vi "InitConnection.vi"(8 "ErrorIn":errorcluster) -> (0 "ErrorOut":errorcluster, 3 "Reference":T1)   [LabVIEW 2022 SP3]
uses:
  C:/Users/Robots/Documents/robocadSimLV/assemblies/LibraryForLabVIEW.dll
  assemblies/LibraryForLabVIEW.dll
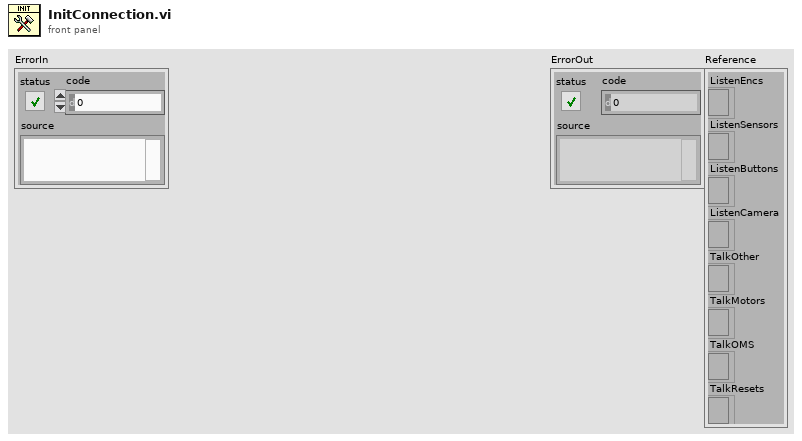
[diagram p1: front panel]
types:
  T1 = cluster{"ListenEncs":refnum<k24>, "ListenSensors":refnum<k24>, "ListenButtons":refnum<k24>, "ListenCamera":refnum<k24>, "TalkOther":refnum<k24>, "TalkMotors":refnum<k24>, "TalkOMS":refnum<k24>, "TalkResets":refnum<k24>}
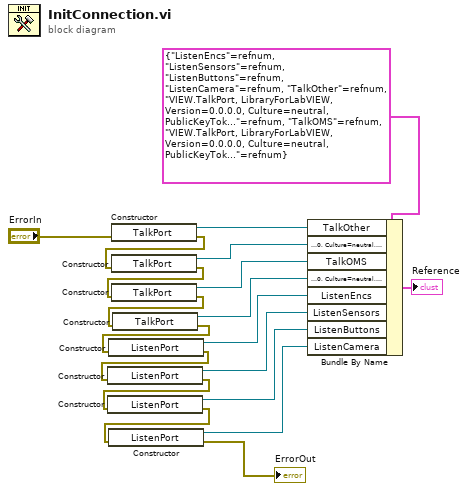
[diagram p0: block diagram]
diagram:
  n1 = constructor class="TalkPort"(error in="ErrorIn") -> (reference out=w17:refnum<k24>, error out=w15:errorcluster)  [unwired: 2 in, 1 out]
  n2 = constructor class="TalkPort"(error in=w15) -> (reference out=w16:refnum<k24>, error out=w13:errorcluster)  [unwired: 2 in, 1 out]
  n3 = constructor class="TalkPort"(error in=w13) -> (reference out=w14:refnum<k24>, error out=w11:errorcluster)  [unwired: 2 in, 1 out]
  n4 = constructor class="TalkPort"(error in=w11) -> (reference out=w12:refnum<k24>, error out=w9:errorcluster)  [unwired: 2 in, 1 out]
  n5 = constructor class="ListenPort"(error in=w9) -> (reference out=w10:refnum<k24>, error out=w7:errorcluster)  [unwired: 2 in, 1 out]
  n6 = constructor class="ListenPort"(error in=w7) -> (reference out=w8:refnum<k24>, error out=w6:errorcluster)  [unwired: 2 in, 1 out]
  n7 = constructor class="ListenPort"(error in=w6) -> (reference out=w5:refnum<k24>, error out=w3:errorcluster)  [unwired: 2 in, 1 out]
  n8 = constructor class="ListenPort"(error in=w3) -> (reference out=w4:refnum<k24>, error out=→"ErrorOut":errorcluster)  [unwired: 2 in, 1 out]
  n9 = Bundle By Name(cluster=T1 {"ListenEncs"=refnum, "ListenSensors"=refnum, "ListenButtons"=refnum, "ListenCamera"=refnum, "TalkOther"=refnum, "TalkMotors"=refnum, "TalkOMS"=refnum, "TalkResets"=refnum}, "TalkOther"=w17, "TalkMotors"=w16, "TalkOMS"=w14, "TalkResets"=w12, "ListenEncs"=w10, "ListenSensors"=w8, "ListenButtons"=w5, "ListenCamera"=w4) -> (→"Reference":T1)
